vi "GEOM_VAR_FPAReadModesUnBin.vi"(9 "Action":T6, 10 "GEOM_FPAReadModes":T1[](array[typedef]) {"Amplifiers"."fliped" items=["none", "horizontal", "vertical"]; "Amplifiers"."type" items=["LL", "LR", "UL", "UR"]}) -> (2 "GEOM_FPAReadModes out":T1[](array[typedef]) {"Amplifiers"."fliped" items=["none", "horizontal", "vertical"]; "Amplifiers"."type" items=["LL", "LR", "UL", "UR"]})   [LabVIEW 2016]
uses:
  GEOM_VAR_action.ctl
  GEOM_FPAReadMode.ctl
  GEOM_Amplifier.ctl
  GEOM_AmpType.ctl
  GEOM_ROI.ctl
  GEOM_Coords.ctl
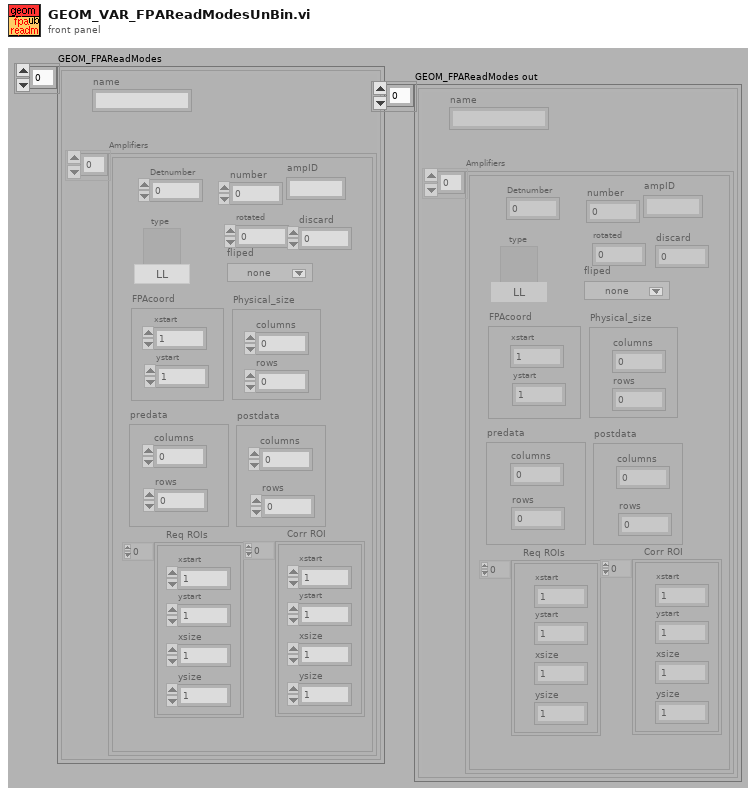
[diagram p1: front panel]
types:
  T1 = typedef "GEOM_FPAReadMode.ctl" = cluster{"name":string, "Amplifiers":T2[]}
  T2 = typedef "GEOM_Amplifier.ctl" = cluster{"number":i32, "type":T3, "rotated":i16, "fliped":u16, "FPAcoord":cluster{"xstart":i32, "ystart":i32}, "Physical_size":cluster{"columns":i32, "rows":i32}, "predata":cluster{"columns":i32, "rows":i32}, "postdata":cluster{"columns":i32, "rows":i32}, "Req ROIs":T4, "Corr ROI":T4, "Detnumber":i32, "ampID":string, "discard":i32}
  T3 = typedef "GEOM_AmpType.ctl" = u16
  T4 = typedef "GEOM_ROI.ctl" = T5[]
  T5 = typedef "GEOM_Coords.ctl" = cluster{"xstart":u32, "ystart":u32, "xsize":u32, "ysize":u32}
  T6 = typedef "GEOM_VAR_action.ctl" = enum16{"read", "write"}
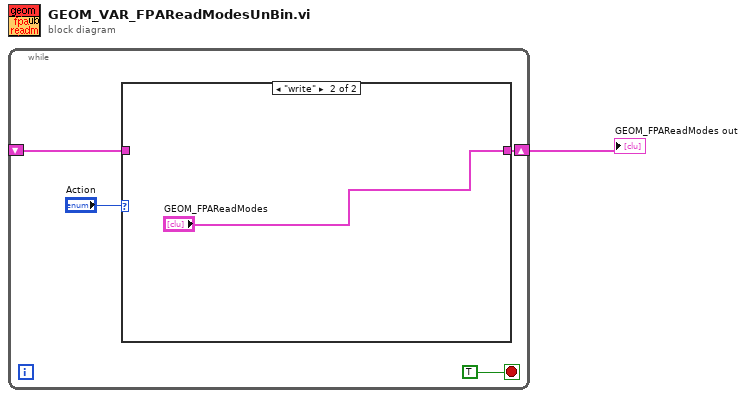
[diagram p0: block diagram]
diagram:
  n1 = while {
    shift-right: [w4] -> w1
    shift-left: _ -> [w3]
    stop <- TRUE stop-if-true
    n2 = case shown="\"write\"" "Action" {
      tunnel: [w6 "GEOM_FPAReadModes"] -> w4
      tunnel: w3 -> [w6 _]
      frame "read", Default {
      }
      frame "write" {
      }
    }
  }
  "GEOM_FPAReadModes out" <- w1
